vi "LfromSpaceCharge_swabish.vi"() -> ()   [LabVIEW 2018]
panel:
  out "center (m)":dbl=-0.36889517 format="%.3f"
  out "x*y":dbl=0.17752047569005144 format="%.3f"
  out "\\phi_0 (v)":dbl=11.937031200000007 format="%.3f"
  out "length (m)":dbl=0.014871409206842934 format="%.3f"
  in  "XY Graph":cluster{"z (mm)":dbl[], "B (T)":dbl[]}[](graph)=[{"z (mm)"=[-0.4946205487469375, -0.48862344329172347, -0.4826232674243275, -0.47662616196911345, -0.4706261041944937, -0.46462616451265015, -0.4586294133357648, -0.45263065458168356, -0.44663248629148344, -0.44063337325907354, -0.43463461450499224, -0.4286382176064356, -0.4226392226668019, -0.41664294386102146, -0.41064583840580743, -0.40464908722892207, -0.39865198177370803, -0.39265499441127016, -0.38666025081158073, -0.38066468056245767, -0.3746691103133346, -0.3686741305280926, -0.36267879646452206, -0.35668558807092354, -0.3506907263784579, -0.34469716370653064, -0.3387039553129322, -0.3327108650121099, -0.32671895563904985, -0.3207259834310039, -0.31473466452182497, -0.30874240087043636, -0.30275084577570505, -0.29675893640264506, -0.2907672632151375, -0.27932879690964096, -0.27333676944380475, -0.2673437972357587, -0.26135212404825114, -0.25535820709799534, -0.24936358159108207, -0.24336860180584013, -0.23846095282252422, -0.22755586097606212, -0.22155568510866613, -0.21555255692186442, -0.2095481297145242, -0.2035415768372119, -0.19753218973327014, -0.191521621701566, -0.18550751088657502, -0.1794919829582694, -0.1734727941539006, -0.1674510073084548, -0.1614294566485614, -0.15567689771436144, -0.14992296890395718, -0.14444164020963107, -0.13896006220833296, -0.13347473148103467, -0.12799089659556862, -0.12277913762546849, -0.11674395315455954, -0.11180517449366983, -0.1068667205879148, -0.10192920847205011, -0.0969905272377008, -0.09178035792758288, -0.08629198303094182, -0.08080810878121703, -0.07532222695429636, -0.06983831334031282, -0.06435743077425249, -0.05832855836223294, -0.05230381919738142, -0.04627778101199137, -0.04025717509430787, -0.034235860619966973, -0.028220332691661243, -0.02220456857780312, -0.01619388245332276, -0.010184022978276086, -0.004177470100963698, 0.0018263666424952474, 0.007827014880996241, 0.01382577363507742, 0.019820517234766966, 0.02581372562836548, 0.03180303696034836, 0.03779199401400268, 0.0437766997277127, 0.049760106420884354, 0.055740915072978736, 0.06171806284901016, 0.06769662773835639, 0.07312683538199505, 0.07855809273920022, 0.08371544046265322, 0.0888723158150011, 0.09429913813238788, 0.09945541252371903, 0.10460888680411173, 0.10976560863585061, 0.11464739277061287, 0.11980353004310951, 0.12522982750371303, 0.13052239801665744, 0.13581343857207862, 0.14151547741660808, 0.14748849194547142, 0.15346292358764968, 0.15943900852869497, 0.16541816388192232, 0.17139850016291192, 0.1773830877838456, 0.18336708494089837, 0.18935533343789523, 0.19534476286265445, 0.20133643605016194, 0.20733070727874647, 0.2133272222700795, 0.21932574483860823, 0.22532556642767554, 0.23132704131561, 0.23733087805906905, 0.24333483289530444, 0.24934114958706421, 0.2553479386499291, 0.2613552000838988, 0.26736387863118316, 0.2733723209929152, 0.27938229856073815, 0.2842985008351323], "B (T)"=[2.701596070156169, 2.9904155729783177, 3.076280830574092, 3.3651003333962404, 3.458771523500719, 3.5602486461139016, 3.872485946462163, 4.052022394162416, 4.270588504406199, 4.426707154580338, 4.606243602280591, 4.941898700154974, 5.105823282837809, 5.449284313220906, 5.738103816043045, 6.050341116391316, 6.339160619213455, 6.635786054544308, 7.080724207540587, 7.471020832975919, 7.86131745841125, 8.290643746390112, 8.69655223684286, 9.242967512452323, 9.680099732939889, 10.203097211023229, 10.7495124866327, 11.303733694750866, 11.936014227956102, 12.498041368582982, 13.16935156433174, 13.778214300010863, 14.433912630742212, 15.066193163947457, 15.71408556217011, 16.963034763563165, 17.587509364259688, 18.14953650488656, 18.79742890310922, 19.29700858366644, 19.749752669171432, 20.179078957150296, 20.354154871988428, 20.795747625338112, 20.881612882933887, 20.77232982781199, 20.57718151509433, 20.241526417219937, 19.718528939136597, 19.11747213596619, 18.282237357534584, 17.353331388998487, 16.182441512692503, 14.83982112119496, 13.512812594714836, 11.934453041454356, 10.26554467109289, 8.583799878383767, 6.885575894822917, 4.939296722652076, 3.0918926955915094, 1.1970025791029748, 1.0312008555073326, 2.9137966282946426, 4.774926086683013, 6.573803233314459, 8.449959111782102, 10.239772703445098, 12.387271469173715, 14.23727747373718, 16.21998433094866, 18.072592313015036, 19.724848027357936, 21.535824369377863, 23.073593073593074, 24.697227035404048, 25.96178810181452, 27.27318476327723, 28.202090731813314, 29.146608565366815, 29.755471301045937, 30.3096925091641, 30.645347607038488, 30.80146625721262, 30.74682472965167, 30.56728828195142, 30.122350128955144, 29.57593485334568, 28.771923804948898, 27.944494959025995, 26.83605254278966, 25.64174486895755, 24.275706679933894, 22.667684583140325, 21.153333676451243, 19.455977018724703, 17.828006427742224, 16.12631314084418, 14.39339612391131, 12.47226940093519, 10.69962886079134, 8.741900987607725, 6.998836258413537, 5.114093854186326, 3.332389759074035, 1.376570002725881, 0.4027489463420775, 2.2831980876894953, 4.044216461653711, 5.925446196252011, 7.7130047407458235, 9.39128023011774, 10.8666014742633, 12.263863393321781, 13.380111742066827, 14.535389753355403, 15.409654194330544, 16.205859310218614, 16.85375170844127, 17.329913591472376, 17.657762756838054, 17.852911069555716, 17.96219412467761, 17.96219412467761, 17.806075474503473, 17.642150891820634, 17.32210765896366, 16.970840696071868, 16.588350003145244, 16.112188120114148, 15.65163810210045, 15.08961096147357, 14.699314336038247]}, {"z (mm)"=array[972 elements], "B (T)"=array[972 elements]}]
  # "0.175"
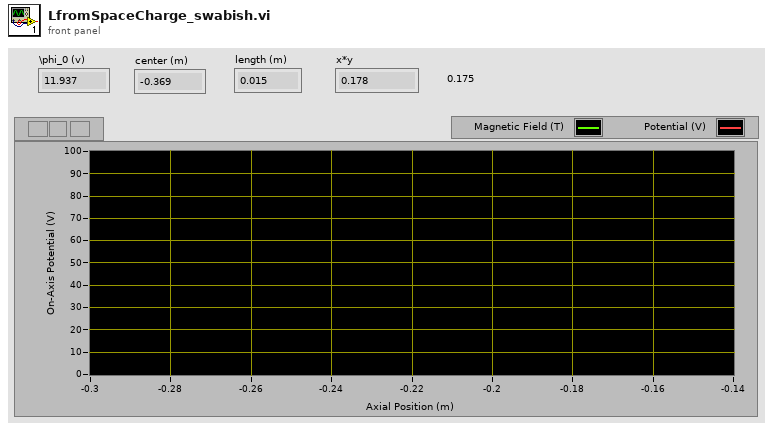
[diagram p1: front panel]
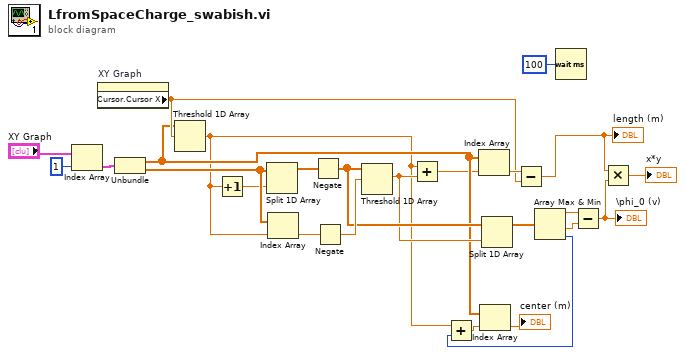
[diagram p0: block diagram]
diagram:
  n1 = Index Array(array="XY Graph", index=1) -> (element=w24:cluster{"z (mm)":dbl[], "B (T)":dbl[]})
  n2 = property on="XY Graph" class="XYGraph (strict)"() -> ("Cursor.Cursor X"=w18:dbl)  [unwired: 2 in, 2 out]
  n3 = Unbundle(w24) -> ("z (mm)"=w6:dbl[], "B (T)"=w22:dbl[])
  n4 = Threshold 1D Array(2:w18, 3:w6) -> (0:w1:dbl)  [unwired: 1 in]
  n5 = Increment(x=w1) -> (x+1=w16:dbl)
  n6 = Split 1D Array(array=w22, index=w16) -> (second subarray=w21:dbl[])  [unwired: 1 out]
  n7 = Index Array(array=w22, index=w1) -> (element=w20:dbl)
  n8 = Negate(x=w21) -> (-x=w15:dbl[])
  n9 = Negate(x=w20) -> (-x=w17:dbl)
  n10 = Threshold 1D Array(2:w17, 3:w15) -> (0:w14:dbl)  [unwired: 1 in]
  n11 = Add(x=w1, y=w14) -> (x+y=w4:dbl)
  n12 = Index Array(array=w6, index=w4) -> (element=w19:dbl)
  n13 = Split 1D Array(array=w15, index=w14) -> (first subarray=w13:dbl[])  [unwired: 1 out]
  n14 = Subtract(x=w19, y=w18) -> (x-y=w9:dbl)
  "length (m)" <- w9
  n15 = Array Max & Min(array=w13) -> (max value=w12:dbl, min value=w11:dbl, min index (indices)=w3:i32)  [unwired: 1 out]
  n16 = Add(x=w1, y=w3) -> (x+y=w5:dbl)
  n17 = Index Array(array=w6, index=w5) -> (element=→"center (m)":dbl)
  n18 = Wait (ms)(milliseconds to wait=u32 100) -> ()  [unwired: 1 out]
  n19 = Subtract(x=w12, y=w11) -> (x-y=w10:dbl)
  "\\phi_0 (v)" <- w10
  n20 = Multiply(x=w9, y=w10) -> (x*y=→"x*y":dbl)
